vi "test Acyclic Loopback Selective Triggers.vi"(8 "error in":errorcluster, 11 "TestCase in":refnum<class "Single Board 1Ch Loopback.lvclass">) -> (0 "error out":errorcluster, 3 "TestCase out":refnum<class "Single Board 1Ch Loopback.lvclass">)   [LabVIEW 2020, in "Single Board 1Ch Loopback.lvclass"]
uses:
  Single Board 1Ch Loopback.lvclass
  C:/dev/git/niveristand-custom-device-testing-tools/VeriStandTestCase/VeriStandTestCase.lvclass
  <vilib>/numeric/Random Number (Range) U64.vi
  <vilib>/numeric/sub_Random U32.vi
  <vilib>/NI VeriStand/Execution/Workspace/NI VeriStand - Set Multiple Channel Values.vi
  <vilib>/addons/_JKI Toolkits/VI Tester/TestCase.llb/TestCase.lvclass
  <vilib>/NI VeriStand/Execution/Workspace/NI_VS Workspace ExecutionAPI.lvlib
  niveristand-custom-device-testing-tools/VeriStandTestUtilities/VeriStandTestUtilities.lvlib
  C:/Program Files (x86)/National Instruments/LabVIEW 2020/vi.lib/addons/_JKI Toolkits/VI Tester/TestCase.llb/TestCase.lvclass
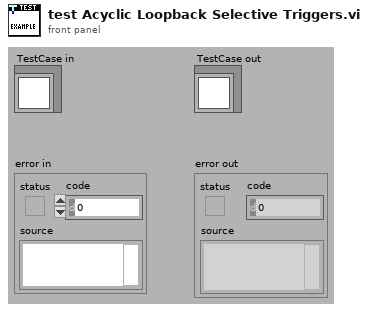
[diagram p1: front panel]
types:
  T1 = typedef "NI_VS Workspace ExecutionAPI.lvlib/WorkspaceAPI.ctl" = refnum<k24>
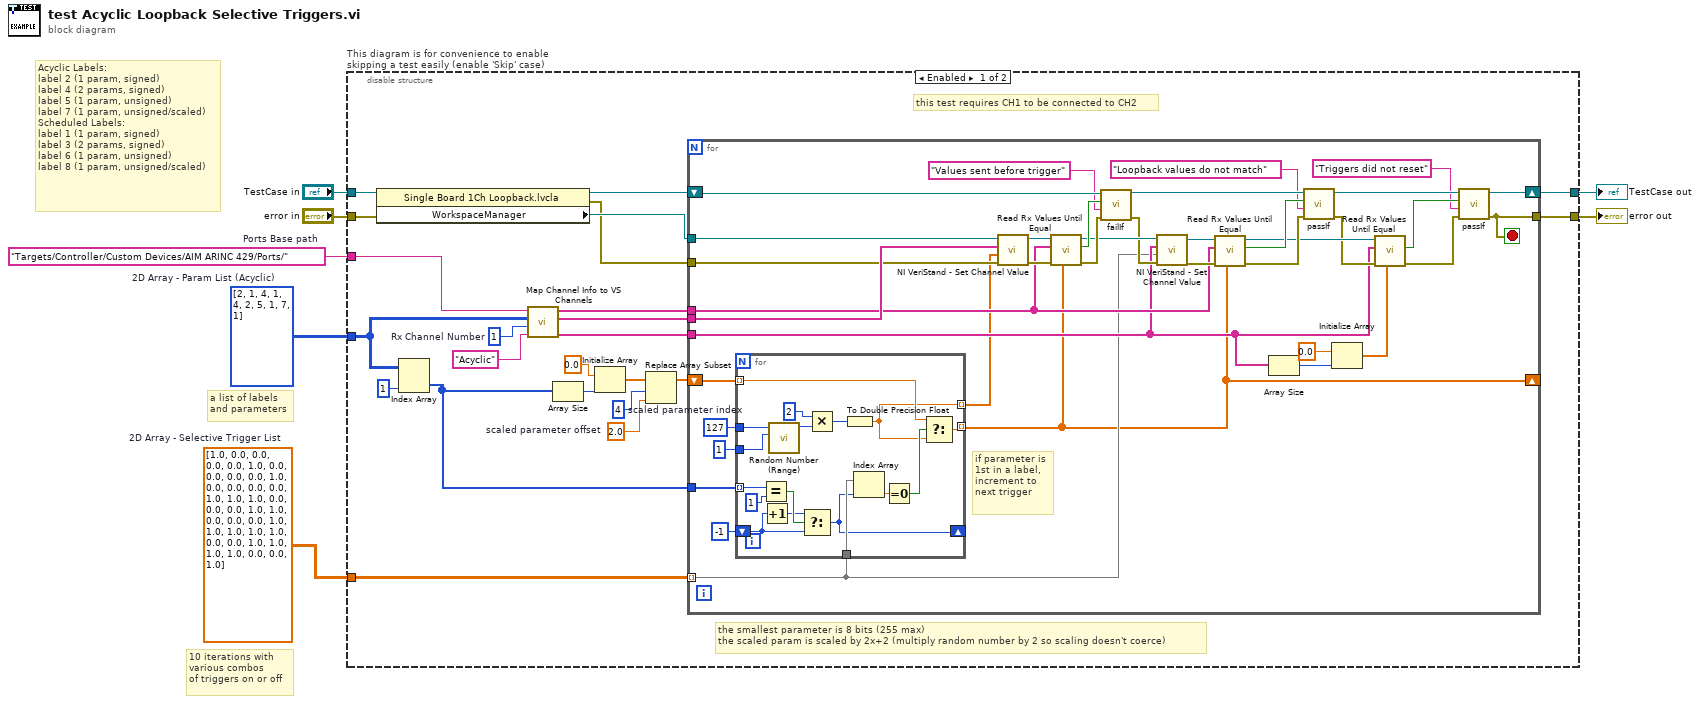
[diagram p0: block diagram]
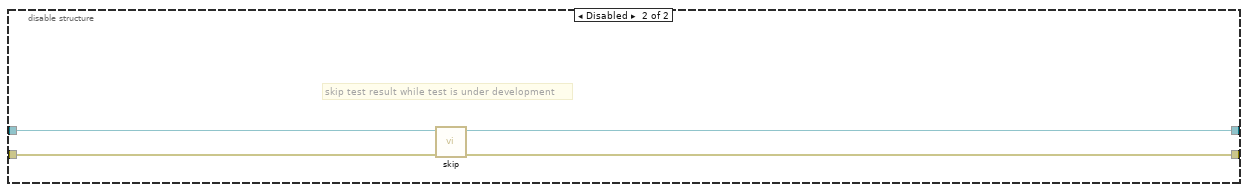
[diagram p2: hidden frame]
diagram:
  w1 = dbl[][] [[1.0, 0.0, 0.0, 0.0], [0.0, 1.0, 0.0, 0.0], [0.0, 0.0, 1.0, 0.0], [0.0, 0.0, 0.0, 1.0], [1.0, 1.0, 0.0, 0.0], [0.0, 1.0, 1.0, 0.0], [0.0, 0.0, 1.0, 1.0], [1.0, 1.0, 1.0, 0.0], [0.0, 1.0, 1.0, 1.0], [1.0, 0.0, 0.0, 1.0]]  # 2D Array - Selective Trigger List
  w3 = i32[][] [[2, 1], [4, 1], [4, 2], [5, 1], [7, 1]]  # 2D Array - Param List (Acyclic)
  w4 = "Targets/Controller/Custom Devices/AIM ARINC 429/Ports/"  # Ports Base path
  # "10 iterations with\nvarious combos\nof triggers on or off"
  # "a list of labels\nand parameters"
  # "Acyclic Labels:\nlabel 2 (1 param, signed)\nlabel 4 (2 params, signed)\nlabel 5 (1 param, unsigned)\nlabel 7 (1 param, unsigned/scaled)\nScheduled Labels:\nlabel 1 (1 param, signed)\nlabel 3 (2 params, signed)\nlabel 6 (1 param, unsigned)\nlabel 8 (1 param, unsigned/scaled)"
  n1 = disable-structure "This diagram is for convenience to enable skipping a test easily (enable 'Skip' case)" shown="Enabled" {
    disable-tunnel: "TestCase in" -> [w25 w89]
    disable-tunnel: [w23 w87] -> w2
    disable-tunnel: [w22 w88] -> w6
    disable-tunnel: "error in" -> [w24 w86]
    disable-tunnel: w4 -> [w26 _]
    disable-tunnel: w3 -> [w17 _]
    disable-tunnel: w1 -> [w15 _]
    frame Enabled {
      w8 = 2.0  # scaled parameter offset
      w9 = 4  # scaled parameter index
      w20 = 1  # Rx Channel Number
      # "this test requires CH1 to be connected to CH2"
      # "the smallest parameter is 8 bits (255 max)\nthe scaled param is scaled by 2x+2 (multiply random number by 2 so scaling doesn't coerce)"
      n2 = property class="Single Board 1Ch Loopback.lvcla"(reference=w25, error in=w24) -> (reference out=w27:refnum<class "Single Board 1Ch Loopback.lvclass">, error out=w28:errorcluster, "WorkspaceManager"=w29:T1)
      n3 = Index Array(array=w17, index (col)=1 ("disabled index (col)")) -> (element=w12:i32[])  [unwired: 1 in]
      n4 = call "Map Channel Info to VS Channels.vi"("Transfer Type"="Acyclic", "Rx Channel Number"=w20, "2D Array - Label/Param List"=w17, "VS Channel Base Port"=w26) -> ("Tx Trigger Channels Array"=w18:string[], "Tx Channels Array"=w19:string[], "Rx Channels Array"=w30:string[])  [unwired: 4 in, 1 out]
      n5 = Array Size(array=w12) -> (size(s)=w13:i32)
      n6 = Initialize Array(0.0 ("element"), w13) -> (w14:dbl[])
      n7 = Replace Array Subset(array=w14, new element=w8, index=w9) -> (w10:dbl[])
      n8 = for {
        tunnel: w30 -> [w54]
        tunnel: w29 -> [w66]
        tunnel: w28 -> [w59]
        tunnel: w19 -> [w65]
        shift-right: [w48] -> w23
        shift-left: w27 -> [w61]
        tunnel: [w50] -> w22
        tunnel: w18 -> [w40]
        tunnel: w15 -> [w35] mode=indexing
        tunnel: w12 -> [w36]
        shift-right: [w32] -> _
        shift-left: w10 -> [w33]
        stop <- w50 stop-if-true
        # "if parameter is 1st in a label, increment to next trigger"
        n9 = for {
          tunnel: [w72] -> w32 mode=indexing
          tunnel: u64 127 ("upper bound (100)") -> [w84]
          tunnel: u64 1 ("upper bound (100)") -> [w83]
          tunnel: w36 -> [w80] mode=indexing
          tunnel: w35 -> [w78]
          shift-right: [w77] -> _
          shift-left: -1 -> [w74]
          tunnel: w33 -> [w70] mode=indexing
          tunnel: [w69] -> w31 mode=indexing
          n10 = Equal?(x=w80, y=1) -> (x = y?=w76:bool)
          n11 = Increment(x=w74) -> (x+1=w75:i32)
          n12 = call-poly <vilib>:"Random Number (Range).vi"("lower bound (0)"=w83, "upper bound (100)"=w84) -> ("number"=w85:u64)  [unwired: 9 in]
          n13 = Select(t=w75, s=w76, f=w74) -> (s? t:f=w77:i32)
          n14 = Multiply(x=u64 2, y=w85) -> (x*y=w82:u64)
          n15 = To Double Precision Float(number=w82) -> (double precision float=w69:dbl)
          n16 = Index Array(array=w78, index=w77) -> (element=w73:dbl)
          n17 = Equal To 0?(x=w73) -> (x = 0?=w71:bool)
          n18 = Select(t=w70, s=w71, f=w69) -> (s? t:f=w72:dbl)
        }
        n19 = call-poly <vilib>:"NI VeriStand - Set Channel Value.vi"("error in (no error)"=w59, "Values"=w31, "Channels"=w65, "WorkspaceManager in"=w66) -> ("error out"=w62:errorcluster, "WorkspaceManager out"=w64:T1)  [unwired: 6 in]
        n20 = call "Read Rx Values Until Equal.vi"("expected values"=w32, "error in"=w62, "Rx aliases"=w54, "workspace manager in"=w64) -> ("error out"=w63:errorcluster, "values equal expected"=w60:bool, "workspace manager out"=w58:T1)  [unwired: 5 in]
        n21 = call-dynamic "failIf.vi"("error in (no error)"=w63, "message (\"\")"="Values sent before trigger" ("message (\"\")"), "fail"=w60, "TestCase in"=w61) -> ("error out"=w57:errorcluster, "TestCase out"=w51:refnum<class "Single Board 1Ch Loopback.lvclass">)  [unwired: 6 in]
        n22 = call-poly <vilib>:"NI VeriStand - Set Channel Value.vi"("error in (no error)"=w57, "Values"=w35, "Channels"=w40, "WorkspaceManager in"=w58) -> ("error out"=w55:errorcluster, "WorkspaceManager out"=w56:T1)  [unwired: 6 in]
        n23 = call "Read Rx Values Until Equal.vi"("expected values"=w32, "error in"=w55, "Rx aliases"=w54, "workspace manager in"=w56) -> ("error out"=w52:errorcluster, "values equal expected"=w53:bool, "workspace manager out"=w46:T1)  [unwired: 5 in]
        n24 = Array Size(array=w40) -> (size(s)=w37:i32)
        n25 = call-dynamic "passIf.vi"("error in (no error)"=w52, "message (\"\")"="Loopback values do not match" ("message (\"\")"), "pass"=w53, "TestCase in"=w51) -> ("error out"=w45:errorcluster, "TestCase out"=w49:refnum<class "Single Board 1Ch Loopback.lvclass">)  [unwired: 6 in]
        n26 = Initialize Array(0.0, w37) -> (w38:dbl[])
        n27 = call "Read Rx Values Until Equal.vi"("expected values"=w38, "error in"=w45, "Rx aliases"=w40, "workspace manager in"=w46) -> ("error out"=w44:errorcluster, "values equal expected"=w47:bool)  [unwired: 5 in, 1 out]
        n28 = call-dynamic "passIf.vi"("error in (no error)"=w44, "message (\"\")"="Triggers did not reset" ("message (\"\")"), "pass"=w47, "TestCase in"=w49) -> ("error out"=w50:errorcluster, "TestCase out"=w48:refnum<class "Single Board 1Ch Loopback.lvclass">)  [unwired: 6 in]
      }
    }
    frame Disabled {
      # "skip test result while test is under development"
      n29 = call <vilib>:"skip.vi"("error in (no error)"=w86, "TestCase in"=w89) -> ("error out"=w88:errorcluster, "TestCase out"=w87:refnum<class "Single Board 1Ch Loopback.lvclass">)  [unwired: 8 in]
    }
  }
  "error out" <- w6
  "TestCase out" <- w2
